vi "nuevos usuarios.vi"() -> ()   [LabVIEW 2018]
uses:
  <vilib>/RAFA Solutions/Harmony UI Controls Kit/String & Path/String Control.ctl
  <vilib>/RAFA Solutions/Harmony UI Controls Kit/String & Path/Combo Box.ctl
  <vilib>/RAFA Solutions/Harmony UI Controls Kit/Boolean/OK Button.ctl
  <vilib>/RAFA Solutions/Harmony UI Controls Kit/Boolean/Cancel Button.ctl
  <vilib>/RAFA Solutions/Harmony UI Controls Kit/Flat UI Design.lvlib
panel:
  in  "Cancel":T1
  in  "OK":T2
  in  "CATEGORIA":T3
  in  "CONTRASEÑA":T4
  in  "USUARIO":T4
  in  "APELLIDO":T4
  in  "NOMBRE":T4
  # "INGRESO DE USUARIOS"
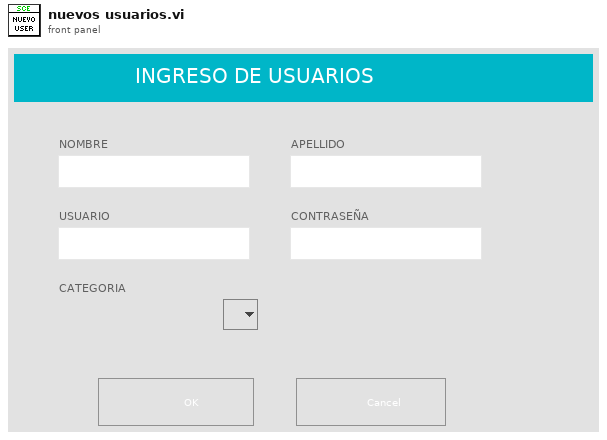
[diagram p1: front panel]
types:
  T1 = typedef "Flat UI Design.lvlib/Cancel Button.ctl" = bool
  T2 = typedef "Flat UI Design.lvlib/OK Button.ctl" = bool
  T3 = typedef "Flat UI Design.lvlib/Combo Box.ctl" = string
  T4 = typedef "Flat UI Design.lvlib/String Control.ctl" = string
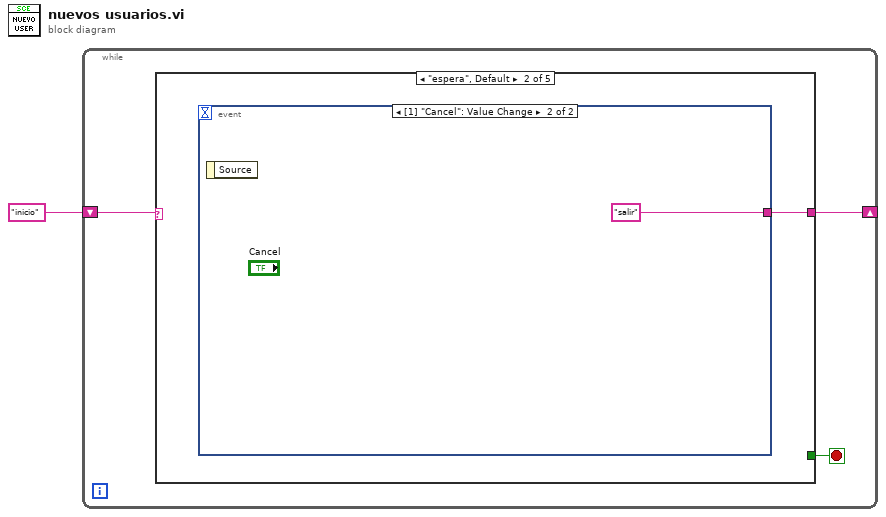
[diagram p0: block diagram]
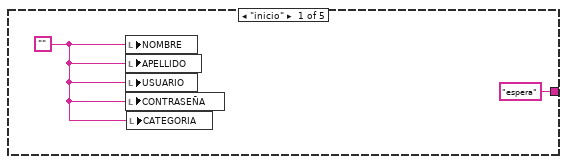
[diagram p2: hidden frame]
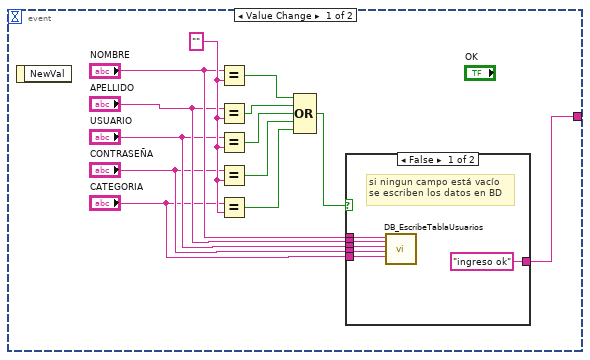
[diagram p3: hidden frame]
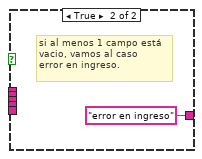
[diagram p4: hidden frame]
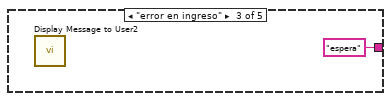
[diagram p5: hidden frame]
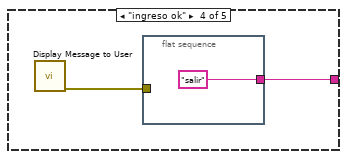
[diagram p6: hidden frame]
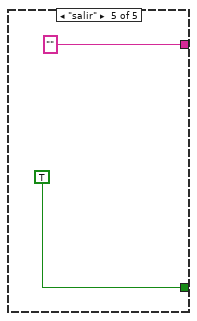
[diagram p7: hidden frame]
diagram:
  n1 = while {
    shift-right: [w3] -> _
    shift-left: "inicio" -> [w4]
    stop <- w2 stop-if-true
    n2 = case shown="\"espera\", Default" w4 {
      tunnel: ["espera" w7 "espera" w31 ""] -> w3
      tunnel: [_ _ _ _ TRUE] -> w2
      frame "inicio" {
        w5 = ""
        n3 = local write "NOMBRE"(w5) -> ()
        n4 = local write "APELLIDO"(w5) -> ()
        n5 = local write "USUARIO"(w5) -> ()
        n6 = local write "CONTRASEÑA"(w5) -> ()
        n7 = local write "CATEGORIA"(w5) -> ()
      }
      frame "espera", Default {
        n8 = event shown="[1] \"Cancel\": Value Change" {
          selector: _ -> [_ _]
          dyn-events: _ -> [_ _]
          timeout: _ -> [_ _]
          tunnel: [w20 "salir"] -> w7
          event Value Change {
            w19 = T4 "" ("y")
            n9 = event-data() -> ()  [unwired: 1 in, 1 out]
            n10 = Equal?(x="NOMBRE", y=w19) -> (x = y?=w18:bool)
            n11 = Equal?(x="APELLIDO", y=w19) -> (x = y?=w17:bool)
            n12 = Equal?(x="USUARIO", y=w19) -> (x = y?=w16:bool)
            n13 = Equal?(x="CONTRASEÑA", y=w19) -> (x = y?=w15:bool)
            n14 = Equal?(x="CATEGORIA", y=w19) -> (x = y?=w14:bool)
            n15 = Compound Arithmetic op=OR(w18, w17, w16, w15, w14) -> (w8:bool)
            n16 = case shown="False" w8 {
              tunnel: ["ingreso ok" "error en ingreso"] -> w20
              tunnel: "NOMBRE" -> [w26 _]
              tunnel: "APELLIDO" -> [w25 _]
              tunnel: "USUARIO" -> [w24 _]
              tunnel: "CONTRASEÑA" -> [w23 _]
              tunnel: "CATEGORIA" -> [w22 _]
              frame False {
                # "si ningun campo está vacío\nse escriben los datos en BD"
                n17 = call "DB_EscribeTablaUsuarios.vi"("NOMBRE"=w26, "APELLIDO"=w25, "USUARIO"=w24, "PASS"=w23, "CATEGORIA"=w22) -> ()  [unwired: 13 in, 2 out]
              }
              frame True {
                # "si al menos 1 campo está\nvacio, vamos al caso\nerror en ingreso."
              }
            }
          }
          event Value Change {
            n18 = event-data() -> ()  [unwired: 1 in, 1 out]
          }
        }
      }
      frame "error en ingreso" {
        n19 = call "Display Message to User2"() -> ()  [unwired: 10 in, 2 out]
      }
      frame "ingreso ok" {
        n20 = call "Display Message to User"() -> ("error out"=w30:errorcluster)  [unwired: 10 in, 1 out]
        n21 = flat-sequence {
          tunnel: ["salir"] -> w31
          tunnel: w30 -> [_]
          frame #0 {
          }
        }
      }
      frame "salir" {
      }
    }
  }
